vi "Song To Song Display.vi"(8 "error in (no error)":errorcluster, 11 "Song":refnum<class "Song.lvclass">) -> (0 "error out":errorcluster, 3 "Song DIsplay":T1 {"Duration (s)" format="%<%M:%S>T"})   [LabVIEW 2015, in "Song.lvclass"]
uses:
  Song.lvclass
  app/controls/Queue Song Display.ctl
  Song Duration.ctl
  app/controls/Dequeue Control.ctl
  MusicElement.lvclass/MusicElement.ctl
  Song.lvclass/Song.ctl
  Read Name.vi
  Read Artist.vi
  Read Album.vi
  Read Duration (s).vi
  Read UID.vi
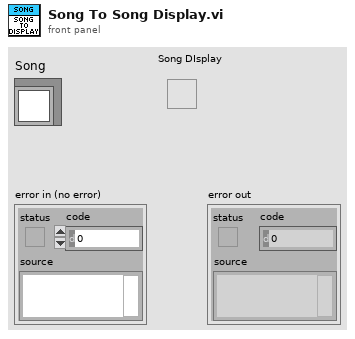
[diagram p1: front panel]
types:
  T1 = typedef "Queue Song Display.ctl" = cluster{"Song Name":string, "Artist":string, "Album":string, "Duration (s)":T2, "UID":string, "Dequeue":T3}
  T2 = typedef "Song.lvclass/Song Duration.ctl" = timestamp
  T3 = typedef "Dequeue Control.ctl" = bool
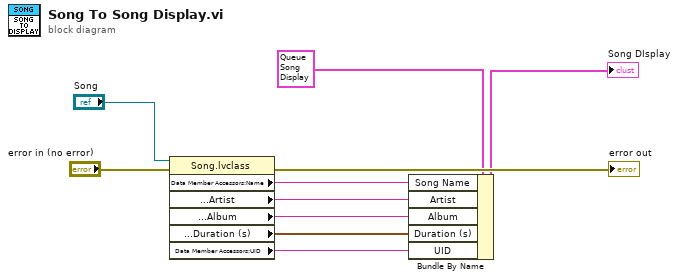
[diagram p0: block diagram]
diagram:
  n1 = property class="Song.lvclass"(reference="Song", error in="error in (no error)") -> (error out=→"error out":errorcluster, "Data Member Accessors:Name"=w8:string, "API:Data Member Accessors:Artist"=w7:string, "API:Data Member Accessors:Album"=w6:string, "API:Data Member Accessors:Duration (s)"=w5:T2, "Data Member Accessors:UID"=w1:string)  [unwired: 1 out]
  n2 = Bundle By Name(cluster=T1 {"Song Name"="", "Artist"="", "Album"="", "Duration (s)"=timestamp(0 s since 1904-01-01), "UID"="", "Dequeue"=FALSE} ("Song"), "Song Name"=w8, "Artist"=w7, "Album"=w6, "Duration (s)"=w5, "UID"=w1) -> (→"Song DIsplay":T1)
